vi "Untitled 1 (SubVI) 1.vi"(6 "collimator afstand\n       (mm)":dbl, 7 "22Na source radius (mm)":dbl, 9 "Numeric":i32, 10 "Array 3":dbl[](array[numeric]), 11 "Array in":i32[](array[numeric])) -> (3 "Array out":dbl[](array[numeric]))   [LabVIEW 2013]
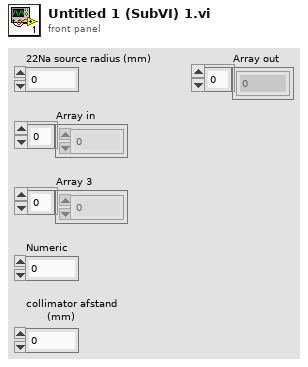
[diagram p1: front panel]
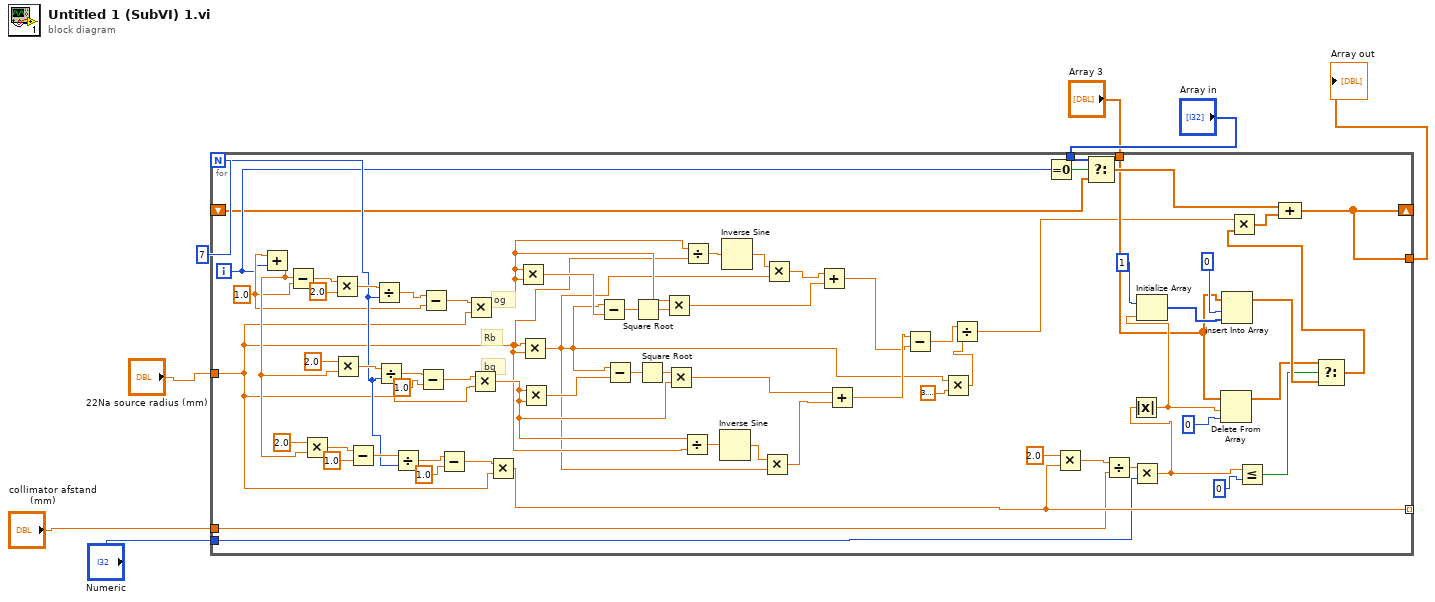
[diagram p0: block diagram]
diagram:
  n1 = for {
    N: 7 -> [w62]
    tunnel: "22Na source radius (mm)" -> [w46]
    tunnel: [w32] -> _ mode=indexing
    tunnel: "collimator afstand\n       (mm)" -> [w30]
    tunnel: "Numeric" -> [w29]
    tunnel: "Array 3" -> [w15]
    tunnel: "Array in" -> [w13]
    shift-right: [w11] -> _
    shift-left: _ -> [w12]
    tunnel: [w11] -> w7
    i -> [w14]
    w57 = 1.0 ("x")
    # "Rb"
    # "bg"
    # "og"
    n2 = Add(x=w57, y=w14) -> (x+y=w58:dbl)
    n3 = Subtract(x=w58, y=w57) -> (x-y=w75:dbl)
    n4 = Multiply(x=2.0, y=w58) -> (x*y=w65:dbl)
    n5 = Multiply(x=w75, y=2.0) -> (x*y=w74:dbl)
    n6 = Multiply(x=2.0, y=w58) -> (x*y=w70:dbl)
    n7 = Subtract(x=w65, y=1.0) -> (x-y=w63:dbl)
    n8 = Divide(x=w74, y=w62) -> (x/y=w73:dbl)
    n9 = Divide(x=w70, y=w62) -> (x/y=w69:dbl)
    n10 = Divide(x=w63, y=w62) -> (x/y=w61:dbl)
    n11 = Subtract(x=w69, y=1.0) -> (x-y=w67:dbl)
    n12 = Subtract(x=w73, y=w57) -> (x-y=w72:dbl)
    n13 = Subtract(x=w61, y=1.0) -> (x-y=w59:dbl)
    n14 = Multiply(x=w72, y=w46) -> (x*y=w47:dbl)
    n15 = Multiply(x=w67, y=w46) -> (x*y=w50:dbl)
    n16 = Multiply(x=w59, y=w46) -> (x*y=w32:dbl)
    n17 = Multiply(x=w47, y=w47) -> (x*y=w53:dbl)
    n18 = Multiply(x=w46, y=w46) -> (x*y=w36:dbl)
    n19 = Multiply(x=w50, y=w50) -> (x*y=w56:dbl)
    n20 = Subtract(x=w36, y=w53) -> (x-y=w52:dbl)
    n21 = Subtract(x=w36, y=w56) -> (x-y=w55:dbl)
    n22 = Square Root(x=w52) -> (sqrt(x)=w51:dbl)
    n23 = Square Root(x=w55) -> (sqrt(x)=w54:dbl)
    n24 = Multiply(x=w47, y=w51) -> (x*y=w40:dbl)
    n25 = Multiply(x=w54, y=w50) -> (x*y=w43:dbl)
    n26 = Divide(x=w50, y=w46) -> (x/y=w49:dbl)
    n27 = Divide(x=w47, y=w46) -> (x/y=w45:dbl)
    n28 = Inverse Sine(1:w49) -> (0:w48:dbl)
    n29 = Inverse Sine(1:w45) -> (0:w44:dbl)
    n30 = Multiply(x=w48, y=w36) -> (x*y=w42:dbl)
    n31 = Multiply(x=w44, y=w36) -> (x*y=w41:dbl)
    n32 = Add(x=w41, y=w40) -> (x+y=w38:dbl)
    n33 = Add(x=w43, y=w42) -> (x+y=w39:dbl)
    n34 = Subtract(x=w39, y=w38) -> (x-y=w35:dbl)
    n35 = Multiply(x=w36, y=3.141592653589793) -> (x*y=w34:dbl)
    n36 = Divide(x=w35, y=w34) -> (x/y=w8:dbl)
    n37 = Equal To 0?(x=w14) -> (x = 0?=w23:bool)
    n38 = Multiply(x=2.0, y=w32) -> (x*y=w31:dbl)
    n39 = Select(t=w13, s=w23, f=w12) -> (s? t:f=w22:dbl[])
    n40 = Divide(x=w31, y=w30) -> (x/y=w28:dbl)
    n41 = Multiply(x=w28, y=w29) -> (x*y=w18:dbl)
    n42 = Absolute Value(x=w18) -> (abs(x)=w17:dbl)
    n43 = Initialize Array(1, w17) -> (w25:i32[])
    n44 = Delete From Array(array=w15, length=w17, index=0) -> (array with subset deleted=w20:dbl[])  [unwired: 1 out]
    n45 = Insert Into Array(array=w15, index=0, new element=w25) -> (w21:dbl[])
    n46 = Less Or Equal?(x=w18, y=0) -> (x <= y?=w16:bool)
    n47 = Select(t=w20, s=w16, f=w21) -> (s? t:f=w9:dbl[])
    n48 = Multiply(x=w8, y=w9) -> (x*y=w10:dbl[])
    n49 = Compound Arithmetic op=ADD(w22, w10) -> (w11:dbl[])
  }
  "Array out" <- w7
